vi "Update Properties Clusters in Compiler.vi"(8 "error in":errorcluster, 10 "Channel Types":string[](array[string]), 11 "VI Path":path) -> (0 "error out":errorcluster)   [LabVIEW 2026, in "NIVS_CDEW_MetaDataObj.lvclass"]
uses:
  NIVS_CDEW_MetaDataObj.lvclass
  NIVS_CDEW_MetaDataObj.lvclass/NIVS_CDEW_MetaDataObj.ctl
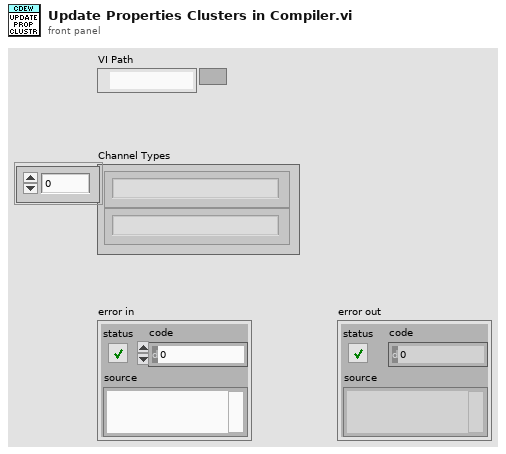
[diagram p1: front panel]
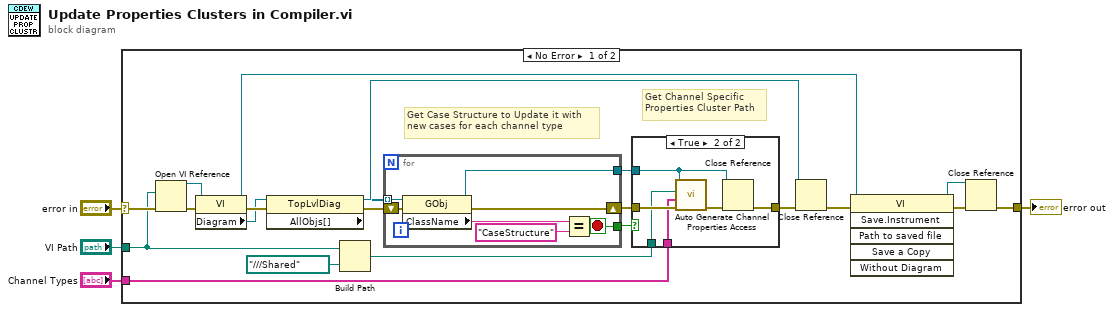
[diagram p0: block diagram]
diagram:
  n1 = case shown="No Error" "error in" {
    selector: "error in" -> [w21 w40]
    tunnel: [w19 w40] -> w3
    tunnel: "Channel Types" -> [w6 _]
    tunnel: "VI Path" -> [w5 _]
    frame No Error {
      # "Get Channel Specific \nProperties Cluster Path"
      # "Get Case Structure to Update it with \nnew cases for each channel type"
      n2 = Open VI Reference(vi path=w5, error in (no error)=w21) -> (vi reference=w14:refnum<vi>, error out=w23:errorcluster)  [unwired: 4 in]
      n3 = property class="VI"(reference=w14, error in=w23) -> (reference out=w16:refnum<vi>, error out=w22:errorcluster, "Diagram"=w13:refnum<vi>)
      n4 = property class="TopLvlDiag"(reference=w13, error in=w22) -> (reference out=w12:refnum<vi>, error out=w20:errorcluster, "AllObjs[]"=w11:refnum<vi>[])
      n5 = Build Path(base path=w5, name or relative path=path "../../../Shared") -> (appended path=w7:path)
      n6 = for {
        tunnel: w11 -> [w37] mode=indexing
        tunnel: [w34] -> w9
        tunnel: [w33] -> w8
        shift-right: [w38] -> w18
        shift-left: w20 -> [w39]
        stop <- w34 stop-if-true
        n7 = property class="GObj"(reference=w37, error in=w39) -> (reference out=w33:refnum<vi>, error out=w38:errorcluster, "ClassName"=w36:string)
        n8 = Equal?(x=w36, y="CaseStructure") -> (x = y?=w34:bool)
      }
      n9 = case shown="True" w9 {
        tunnel: w6 -> [_ w27]
        tunnel: [w26 w32] -> w17
        tunnel: w18 -> [w26 w30]
        tunnel: w8 -> [_ w29]
        tunnel: w7 -> [_ w28]
        frame False {
        }
        frame True {
          n10 = call "Auto Generate Channel Properties Access.vi"("error in"=w30, "Channel Types"=w27, "Path"=w28, "Reference in"=w29) -> ("error out"=w31:errorcluster)  [unwired: 7 in]
          n11 = Close Reference(reference=w29, error in (no error)=w31) -> (error out=w32:errorcluster)
        }
      }
      n12 = Close Reference(reference=w12, error in (no error)=w17) -> (error out=w25:errorcluster)
      n13 = invoke class="VI" method="Save.Instrument"(reference=w16, error in=w25) -> (reference out=w15:refnum<vi>, error out=w24:errorcluster)  [unwired: 4 in, 4 out]
      n14 = Close Reference(reference=w15, error in (no error)=w24) -> (error out=w19:errorcluster)
    }
    frame Error {
    }
  }
  "error out" <- w3
